vi "Lock_1_Plot.vi"(10 "Ось Y":i32[](array[numeric]), 11 "XY Graph ref":refnum<vi>) -> (0 "error out":errorcluster)   [LabVIEW 2023, in "Graph_data_collector.lvlib" / "Graph_UI.lvlib"]
uses:
  Graph_UI.lvlib
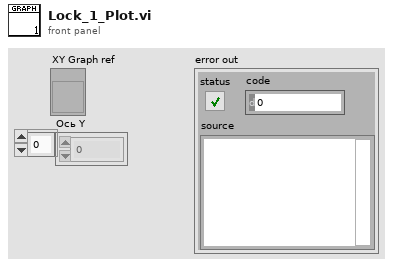
[diagram p1: front panel]
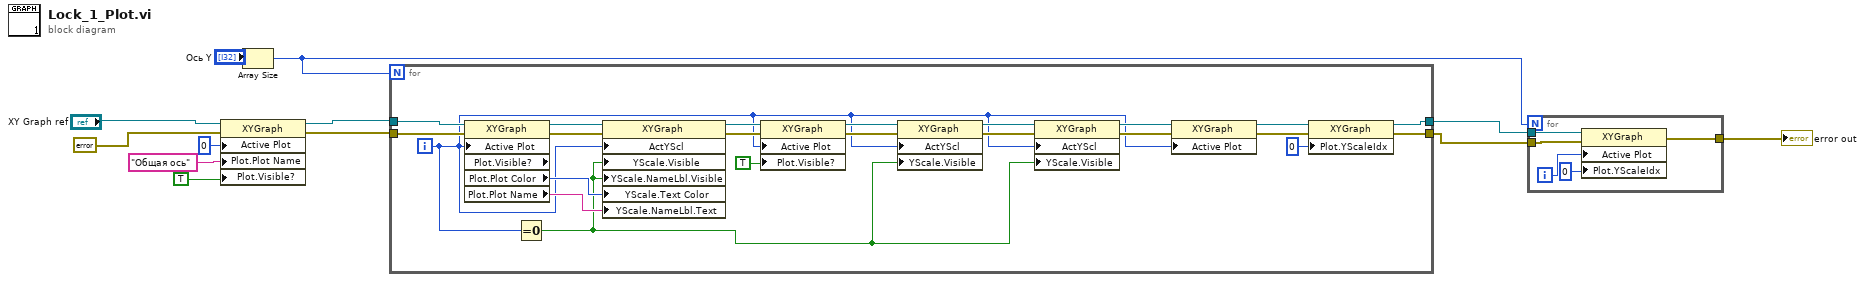
[diagram p0: block diagram]
diagram:
  n1 = property on="Property Node" class="XYGraph"(reference="XY Graph ref", error in=errorcluster {"status"=FALSE, "code"=0, "source"=""} ("error out"), "Active Plot"=u32 0, "Plot.Plot Name"="Общая ось", "Plot.Visible?"=TRUE ("Plot.Visible")) -> (reference out=w9:refnum<vi>, error out=w8:errorcluster)
  n2 = Array Size(array="Ось Y") -> (size(s)=w1:i32)
  n3 = for {
    N: w1 -> [_]
    tunnel: w8 -> [w34]
    tunnel: w9 -> [w29]
    tunnel: [w17] -> w12
    tunnel: [w18] -> w11
    i -> [w15]
    n4 = property on="Property Node" class="XYGraph" props=["Active Plot", "Plot", "Visible?", "Plot", "Plot Color", "Plot", "Plot Name"](reference=w29, error in=w34, "Active Plot"=w15) -> (reference out=w30:refnum<vi>, error out=w31:errorcluster, "Plot.Plot Color"=w32:u32, "Plot.Plot Name"=w33:string)  [unwired: 1 out]
    n5 = Equal To 0?(x=w15) -> (x = 0?=w14:bool)
    n6 = property on="Property Node" class="XYGraph"(reference=w30, error in=w31, "ActYScl"=w15, "YScale.Visible"=w14, "YScale.NameLbl.Visible"=w14, "YScale.Text Color"=w32, "YScale.NameLbl.Text"=w33) -> (reference out=w28:refnum<vi>, error out=w27:errorcluster)
    n7 = property on="Property Node" class="XYGraph"(reference=w28, error in=w27, "Active Plot"=w15, "Plot.Visible?"=TRUE ("Plot.Visible")) -> (reference out=w26:refnum<vi>, error out=w25:errorcluster)
    n8 = property on="Property Node" class="XYGraph"(reference=w26, error in=w25, "ActYScl"=w15, "YScale.Visible"=w14) -> (reference out=w24:refnum<vi>, error out=w23:errorcluster)
    n9 = property on="Property Node" class="XYGraph"(reference=w24, error in=w23, "ActYScl"=w15, "YScale.Visible"=w14) -> (reference out=w22:refnum<vi>, error out=w21:errorcluster)
    n10 = property on="Property Node" class="XYGraph"(reference=w22, error in=w21, "Active Plot"=w15) -> (reference out=w20:refnum<vi>, error out=w19:errorcluster)
    n11 = property on="Property Node" class="XYGraph"(reference=w20, error in=w19, "Plot.YScaleIdx"=u32 0 ("Plot.Y Scale Index")) -> (reference out=w17:refnum<vi>, error out=w18:errorcluster)
  }
  n12 = for {
    N: w1 -> [_]
    tunnel: w12 -> [w39]
    tunnel: [w37] -> w10
    tunnel: w11 -> [w36]
    i -> [w38]
    n13 = property on="Property Node" class="XYGraph"(reference=w39, error in=w36, "Active Plot"=w38, "Plot.YScaleIdx"=u32 0 ("Plot.Y Scale Index")) -> (error out=w37:errorcluster)  [unwired: 1 out]
  }
  "error out" <- w10
